vi "Error Handle_SubVIs-某型振动实验台测试系统.vi"(8 "error in":errorcluster) -> (0 "error out":errorcluster)   [LabVIEW 2015]
doc: "若发生错误，显示错误信息"
uses:
  <vilib>/Utility/error.llb/DialogType.ctl
panel:
  out "Warn":bool
  in  "OK":bool
  out "Hint":string
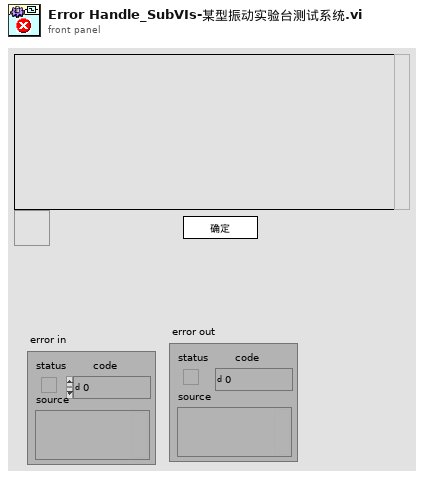
[diagram p1: front panel]
types:
  T1 = typedef "DialogType.ctl" = u16
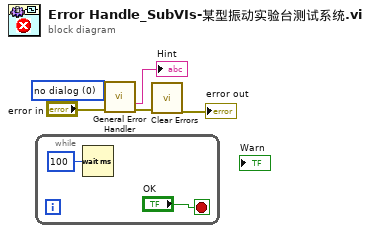
[diagram p0: block diagram]
diagram:
  w2 = T1 0 items=["no dialog", "OK message", "continue or stop message", "OK message + warnings", "continue/stop + warnings"] ("type of dialog (OK msg:1)")
  n1 = while {
    stop <- "OK" stop-if-true
    n2 = Wait (ms)(milliseconds to wait=u32 100) -> ()  [unwired: 1 out]
  }
  n3 = call <vilib>:"General Error Handler.vi"("type of dialog (OK msg:1)"=w2, "error in (no error)"="error in") -> ("message"=→"Hint":string, "error out"=w5:errorcluster)  [unwired: 1 in, 11 out]
  n4 = call <vilib>:"Clear Errors.vi"("error in (no error)"=w5) -> ("error out"=→"error out":errorcluster)  [unwired: 1 in, 5 out]
